vi "Copy Package.vi"(8 "error in (no error)":errorcluster, 11 "PostBuildSupport in":refnum<class "PostBuildSupport.lvclass">) -> (0 "error out":errorcluster, 3 "PostBuildSupport out":refnum<class "PostBuildSupport.lvclass">)   [LabVIEW 2019, in "PostBuildSupport.lvclass"]
uses:
  PostBuildSupport.lvclass
  PostBuildSupport.lvclass/PostBuildSupport.ctl
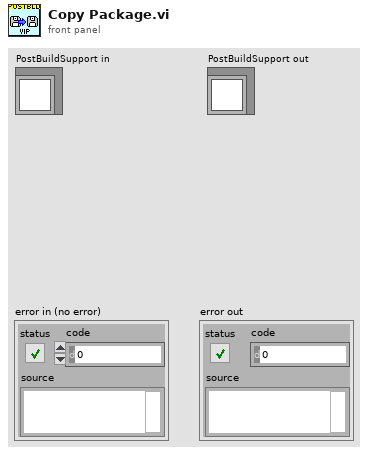
[diagram p1: front panel]
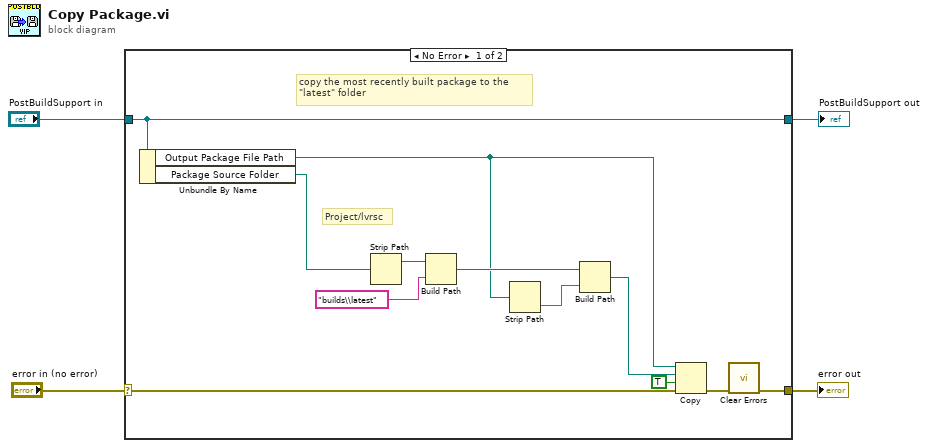
[diagram p0: block diagram]
diagram:
  n1 = case shown="No Error" "error in (no error)" {
    selector: "error in (no error)" -> [w11 w18]
    tunnel: [w8 w18] -> w4
    tunnel: "PostBuildSupport in" -> [w10 w17]
    tunnel: [w10 w17] -> w1
    frame No Error {
      # "Project/lvrsc"
      # "copy the most recently built package to the \n\"latest\" folder"
      n2 = Unbundle By Name(w10) -> ("Output Package File Path"=w5:path, "Package Source Folder"=w12:path)
      n3 = Strip Path(path=w12) -> (stripped path=w16:path)  [unwired: 1 out]
      n4 = Build Path(base path=w16, name or relative path="builds\\latest") -> (appended path=w7:path)
      n5 = Strip Path(path=w5) -> (name=w15:string)  [unwired: 1 out]
      n6 = Build Path(base path=w7, name or relative path=w15) -> (appended path=w14:path)
      n7 = Copy(8:w11, 9:TRUE ("overwrite (F)"), 10:w14, 11:w5) -> (0:w9:errorcluster)  [unwired: 1 in, 2 out]
      n8 = call <vilib>:"Clear Errors.vi"("error in (no error)"=w9) -> ("error out"=w8:errorcluster)  [unwired: 5 in, 1 out]
    }
    frame Error {
    }
  }
  "error out" <- w4
  "PostBuildSupport out" <- w1
